vi "sub_getBooleanDisplayText.vi"(11 "?":refnum<vi>) -> (3 "True Label":string)   [LabVIEW 2018]
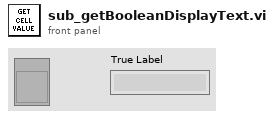
[diagram p1: front panel]
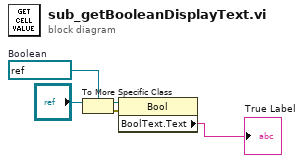
[diagram p0: block diagram]
diagram:
  w5 = refnum<vi> refnum  # Boolean
  n1 = To More Specific Class(target class=w5, reference="?") -> (specific class reference=w4:refnum<vi>, error out=w2:errorcluster)  [unwired: 1 in]
  n2 = property class="Bool"(reference=w4, error in=w2) -> ("BoolText.Text"=→"True Label":string)  [unwired: 2 out]
